vi "ROI entry screen-LBox clear.vi"(8 "error in (no error)":errorcluster, 10 "ROIs for deletion":i32[](array[numeric]), 11 "Function":T1=enum."Clear Last") -> (0 "error out":errorcluster)   [LabVIEW 2020]
uses:
  Typedefs/ROI management FG states.ctl
  Globals/gl_ROI Entry UI globals.vi
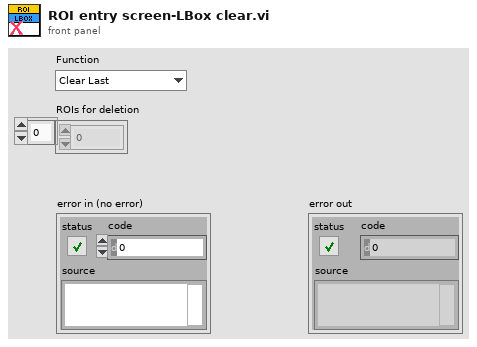
[diagram p1: front panel]
types:
  T1 = typedef "ROI management FG states.ctl" = enum16{"Read", "Write", "Write-from dataset", "Clear Last", "Clear All", "Delete ROI", "Update ROIs time", "Reload last ROI set", "Modify ROI Parameters", "Offset all ROI", "Offset visible ROI", "Modify Dwell Time", "Modify Laser Power"}
  T2 = typedef "ROI entry screen ctrl refs cluster.ctl" = cluster{"Done button":refnum<vi>, "Imaging button":refnum<vi>, "Acquisition button":refnum<vi>, "Scan dwell time per pixel (us)":refnum<vi>, "# of planes":refnum<vi>, "Zoom Ctrl":refnum<vi>, "Equal size":refnum<vi>, "Channel":refnum<vi>, "Image Display":refnum<vi>, "Z-Plane Selector":refnum<vi>, "Number of lines left":refnum<vi>, "Z-stack folder path":refnum<vi>, "POI Density":refnum<vi>, "Arb Plane Entry":refnum<vi>, "Whole Plane":refnum<vi>, "Line Mode":refnum<vi>, "Clear Last":refnum<vi>, "Clear All":refnum<vi>, "Delete Lines":refnum<vi>, "Trial Length (sec)":refnum<vi>, "Palette Type":refnum<vi>, "Intensity slider":refnum<vi>, "# POI":refnum<vi>, "Max Z Proj":refnum<vi>, "Zplane ind":refnum<vi>, "Wavelength (nm)":refnum<vi>, "Number of Trials":refnum<vi>, "Funct stim.trig.enable":refnum<vi>, "Funct stim.trig.delay (s)":refnum<vi>, "Line Mode":refnum<vi>, "Step size (µm)":refnum<vi>, "ROI move mode":refnum<vi>, "Cool-down time (s)":refnum<vi>, "Enable cool-down time":refnum<vi>, "Motor Z ind. (um)":refnum<vi>, "AOL Z ind. (um)":refnum<vi>, "Load Reference Image":refnum<vi>, "Rel.  Res.":refnum<vi>, "ROI LIST":refnum<vi>, "Show All":refnum<vi>, "ROI Type":refnum<vi>, "Start Plane":refnum<vi>, "Stop Plane":refnum<vi>, "Offset ROI":refnum<vi>, "Tab Control":refnum<vi>, "Laser Power(%)":refnum<vi>, "Cycle rate":refnum<vi>, "FOV (Ind.)":refnum<vi>, "Frame Size (Ind.)":refnum<vi>, "Resolution (Ind.)":refnum<vi>, "Pixel Density (Ind)":refnum<vi>, "Laser Power (Ind.)":refnum<vi>, "Dwell Time (Ind.)":refnum<vi>, "Adj MC":refnum<vi>}
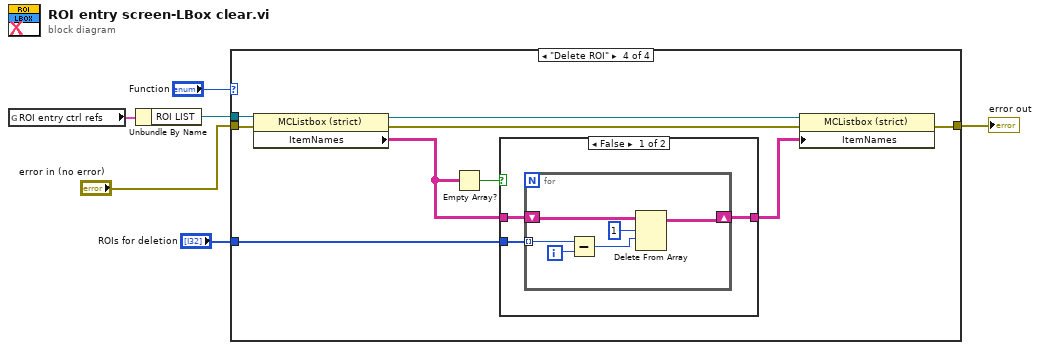
[diagram p0: block diagram]
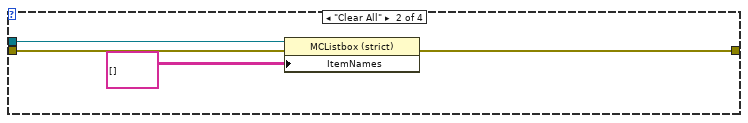
[diagram p3: hidden frame]
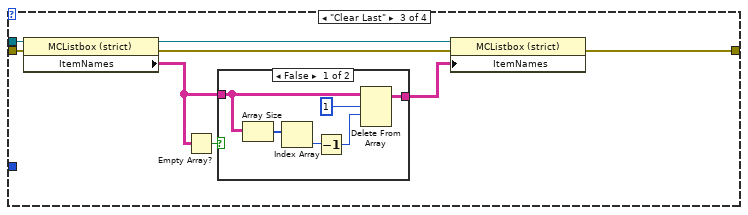
[diagram p4: hidden frame]
diagram:
  n1 = global read "gl_ROI Entry UI globals.vi" "ROI entry ctrl refs"() -> (w6:T2)
  n2 = Unbundle By Name(w6) -> ("ROI LIST"=w5:refnum<vi>)
  n3 = case shown="\"Delete ROI\"" "Function" {
    tunnel: w5 -> [_ w11 w19 w30]
    tunnel: "error in (no error)" -> [w7 w10 w18 w29]
    tunnel: [w7 w9 w12 w28] -> w3
    tunnel: "ROIs for deletion" -> [_ _ _ w27]
    frame Default {
    }
    frame "Clear All" {
      n4 = property class="MCListbox (strict)"(reference=w11, error in=w10, "ItemNames"=string[][] [] ("Item Names")) -> (error out=w9:errorcluster)  [unwired: 1 out]
    }
    frame "Clear Last" {
      n5 = property class="MCListbox (strict)"(reference=w19, error in=w18) -> (reference out=w16:refnum<vi>, error out=w17:errorcluster, "ItemNames"=w15:string[][])
      n6 = Empty Array?(array=w15) -> (empty?=w14:bool)
      n7 = case shown="False" w14 {
        tunnel: w15 -> [w23 w26]
        tunnel: [w20 w26] -> w13
        frame False {
          n8 = Array Size(array=w23) -> (size(s)=w25:i32[])
          n9 = Index Array(array=w25) -> (element=w24:i32)  [unwired: 1 in]
          n10 = Decrement(x=w24) -> (x-1=w22:i32)
          n11 = Delete From Array(array=w23, length=1, index (row)=w22) -> (array with subset deleted=w20:string[][])  [unwired: 1 in, 1 out]
        }
        frame True {
        }
      }
      n12 = property class="MCListbox (strict)"(reference=w16, error in=w17, "ItemNames"=w13) -> (error out=w12:errorcluster)  [unwired: 1 out]
    }
    frame "Delete ROI" {
      n13 = property class="MCListbox (strict)"(reference=w30, error in=w29) -> (reference out=w34:refnum<vi>, error out=w35:errorcluster, "ItemNames"=w33:string[][])
      n14 = Empty Array?(array=w33) -> (empty?=w32:bool)
      n15 = case shown="False" w32 {
        tunnel: w33 -> [w38 w45]
        tunnel: [w36 w45] -> w31
        tunnel: w27 -> [w37 _]
        frame False {
          n16 = for {
            shift-right: [w41] -> w36
            shift-left: w38 -> [w42]
            tunnel: w37 -> [w40] mode=indexing
            i -> [w39]
            n17 = Subtract(x=w40, y=w39) -> (x-y=w44:i32)
            n18 = Delete From Array(array=w42, length=1, index (row)=w44) -> (array with subset deleted=w41:string[][])  [unwired: 1 in, 1 out]
          }
        }
        frame True {
        }
      }
      n19 = property class="MCListbox (strict)"(reference=w34, error in=w35, "ItemNames"=w31) -> (error out=w28:errorcluster)  [unwired: 1 out]
    }
  }
  "error out" <- w3
